vi "Add To DAQmx Task.vi"(6 "Ignore Cal? (F)":bool, 7 "Dynamic in":refnum<class "Dynamic.lvclass">, 8 "error in (no error)":errorcluster, 9 "Scale Name":string, 10 "Chassis Name":string, 11 "task in":refnum<k21>) -> (0 "error out":errorcluster, 2 "Phys Chan Added":string, 3 "task out":refnum<k21>)   [LabVIEW 2018, in "Measurement Channels.lvlib" / "Dynamic.lvclass"]
uses:
  Dynamic.lvclass
  C:/Users/Jeff Tipps/Documents/DAQMan/source/Classes/Measurements/Class Channel/Channel.lvclass
  C:/Users/Jeff Tipps/Documents/DAQMan/source/Classes/Measurements/Class Voltage/Voltage.lvclass
  Dynamic.lvclass/Dynamic.ctl
  Class Channel/Read ChanName.vi
  Class Channel/Read Alias.vi
  Class Channel/Read Unit_EU.vi
  Class Voltage/Read VRange.vi
  <vilib>/DAQmx/create/scale.llb/DAQmx Create Scale (Linear).vi
  <vilib>/DAQmx/create/channels.llb/DAQmx Create Channel (AI-Voltage-Basic).vi
  <resource>/objmgr/daqmx.rc
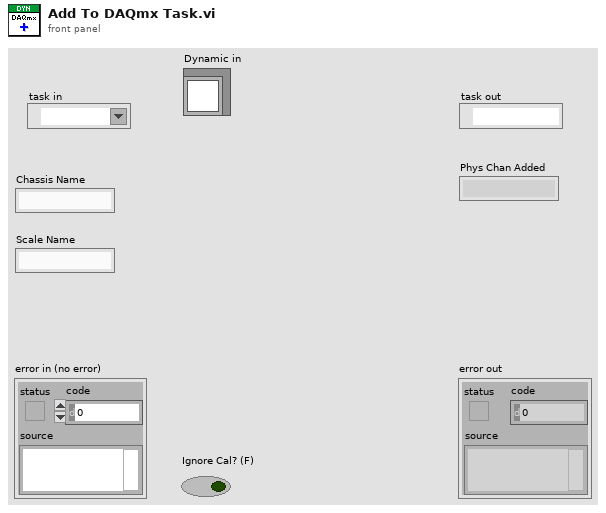
[diagram p1: front panel]
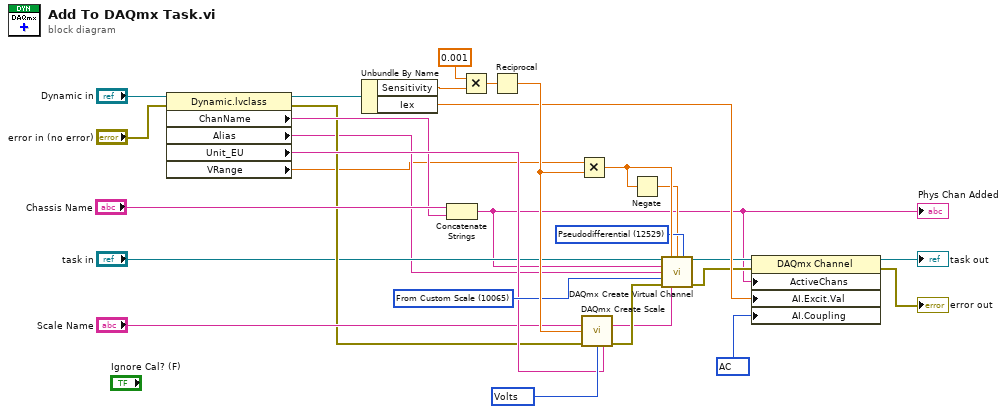
[diagram p0: block diagram]
diagram:
  w23 = 10065 items=["Volts"=10348, "From Custom Scale"=10065] ("units")
  w21 = 12529 items=["default"=-1, "RSE"=10083, "NRSE"=10078, "Differential"=10106, "Pseudodifferential"=12529] ("input terminal configuration")
  w18 = 10045 items=["AC"=10045, "DC"=10050, "GND"=10066] ("AI.Coupling")
  w22 = 10348 items=["Volts"=10348, "Amps"=10342, "Deg F"=10144, "Deg C"=10143, "Deg R"=10145, "Kelvins"=10325, "Strain"=10299, "Ohms"=10384, "Hz"=10373, "Seconds"=10364, "Meters"=10219, "Inches"=10379, "Degrees"=10146, "Radians"=10273, "g"=10186, "m/s^2"=12470, "Pascals"=10081, "Newtons"=15875, "Pounds"=15876, "kgf"=15877, "psi"=15879, "bar"=15880, "Nm"=15881, "oz-in"=15882, "lb-in"=15883, "lb-ft"=15884, "Volts/Volt"=15896, "mVolts/Volt"=15897, "From TEDS"=12516] ("pre-scaled units")
  n1 = property class="Dynamic.lvclass"(reference="Dynamic in", error in="error in (no error)") -> (reference out=w14:refnum<class "Dynamic.lvclass">, error out=w9:errorcluster, "ChanName"=w11:string, "Alias"=w6:string, "Unit_EU"=w13:string, "VRange"=w5:dbl)
  n2 = Unbundle By Name(w14) -> ("Sensitivity"=w24:dbl, "Iex"=w26:dbl)
  n3 = Concatenate Strings("Chassis Name", w11) -> (w1:string)
  "Phys Chan Added" <- w1
  n4 = Multiply(x=0.001, y=w24) -> (x*y=w28:dbl)
  n5 = Reciprocal(x=w28) -> (1/x=w29:dbl)
  n6 = Multiply(x=w5, y=w29) -> (x*y=w27:dbl)
  n7 = call-poly <vilib>:"DAQmx Create Scale.vi"("name"="Scale Name", "slope"=w29, "error in"=w9, "pre-scaled units"=w22, "scaled units"=w13) -> ("scale out"=w2:tag, "error out"=w16:errorcluster)  [unwired: 9 in]
  n8 = Negate(x=w27) -> (-x=w20:dbl)
  n9 = call-poly <vilib>:"DAQmx Create Virtual Channel.vi"("task in"="task in", "maximum value"=w27, "minimum value"=w20, "input terminal configuration"=w21, "physical channels"=w1, "name to assign"=w6, "units"=w23, "error in"=w16, "custom scale name"=w2) -> ("task out"=w17:refnum<k21>, "error out"=w19:errorcluster)  [unwired: 5 in]
  n10 = property class="DAQmx Channel"(reference=w17, error in=w19, "ActiveChans"=w1, "AI.Excit.Val"=w26, "AI.Coupling"=w18) -> (reference out=→"task out":refnum<k21>, error out=→"error out":errorcluster)
